vi "Swerve Drive.vi"(0 "X":dbl(slide) scale=-1.0..1.0, 1 "Rot. Point Y":dbl, 3 "Rot. Point X":dbl, 7 "Y":dbl(slide) scale=1.0..-1.0, 11 "Z":dbl(knob) scale=1.0..-1.0, 12 "Auto Controls":bool, 13 "Robot-Centric":bool) -> ()   [LabVIEW 2020]
uses:
  <vilib>/Rock Robotics/Network Tables/NT Write Boolean.vi
panel:
  in  "Robot Length":dbl=21.5
  in  "Robot Width":dbl=29.5
  # "SWERVE DRIVE\nVersion 3.1\n\nCory Lynch\nApple Pi Robotics\nTeam 2067"
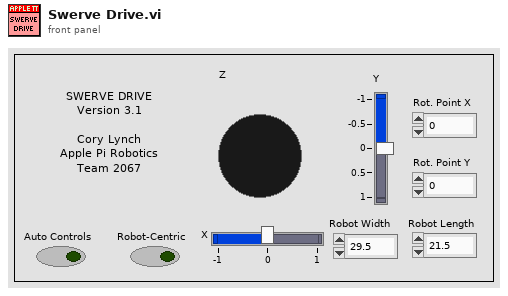
[diagram p1: front panel]
types:
  T1 = enum16{"Back Left", "Back Right", "Front Left", "Front Right"}
  T2 = cluster{"Yaw":dbl, "Roll":dbl, "Pitch":dbl, "Heading":dbl, "Fused Heading":dbl}
  T3 = typedef "WPI_MotorControlDeviceRef.ctl" = cluster{"DeviceStatus":errorcluster, "Type":T4, "PWM":cluster{"PWM Channel":T5, "DeadBand":T6}, "CAN":cluster{"Device Number":u8, "SetOutput VI Ref":variant, "GetOutput VI Ref":variant, "Enable VI Ref":variant, "Disable VI Ref":variant, "Data":variant}, "Invert":bool, "DIO PWM":cluster{"PWM \"Enable\" Channel":T5, "DIOChannel":T7, "PWM Rate":dbl}}
  T4 = typedef "WPI_MotorControlType.ctl" = enum16{"PWM", "CAN", "DIO PWM"}
  T5 = typedef "FPGA_DIOPWMChannel.ctl" = enum8{"PWM 0", "PWM 1", "PWM 2", "PWM 3", "PWM 4", "PWM 5", "PWM 6", "PWM 7", "PWM 8", "PWM 9", "PWM MXP 0", "PWM MXP 1", "PWM MXP 2", "PWM MXP 3", "PWM MXP 4", "PWM MXP 5", "PWM MXP 6", "PWM MXP 7", "PWM MXP 8", "PWM MXP 9", "Invalid"}
  T6 = typedef "WPI_PWMDeadband.ctl" = cluster{"Name":string, "maxPositivePwm":i32, "minPositivePwm":i32, "centerPwm":i32, "maxNegativePwm":i32, "minNegativePwm":i32, "angularRange":u16}
  T7 = typedef "FPGA_DIOChannel.ctl" = enum8{"DIO 0", "DIO 1", "DIO 2", "DIO 3", "DIO 4", "DIO 5", "DIO 6", "DIO 7", "DIO 8", "DIO 9", "DIO MXP 0", "DIO MXP 1", "DIO MXP 2", "DIO MXP 3", "DIO MXP 4", "DIO MXP 5", "DIO MXP 6", "DIO MXP 7", "DIO MXP 8", "DIO MXP 9", "DIO MXP 10", "DIO MXP 11", "DIO MXP 12", "DIO MXP 13", "DIO MXP 14", "DIO MXP 15", "SPI Port CS1", "SPI Port CS2", "SPI Port CS3", "SPI Port MISO", "SPI Port MOSI", "Invalid"}
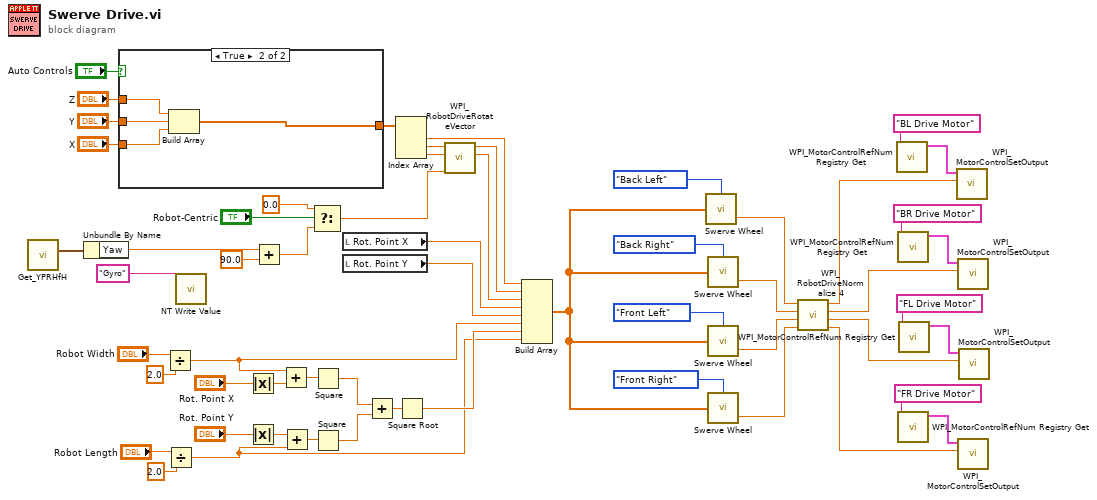
[diagram p0: block diagram]
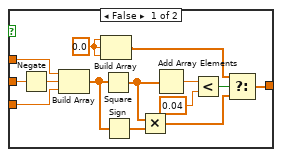
[diagram p2: hidden frame]
diagram:
  n1 = call <vilib>:"Get_YPRHfH.vi"() -> ("YRPHfH"=w6:T2)  [unwired: 11 in]
  n2 = Unbundle By Name(w6) -> ("Yaw"=w3:dbl)
  n3 = case shown="True" "Auto Controls" {
    tunnel: "Y" -> [w68 w74]
    tunnel: "X" -> [w62 w75]
    tunnel: "Z" -> [w58 w72]
    tunnel: [w59 w73] -> w14
    frame False {
      w66 = 0.0 ("element")
      n4 = Negate(x=w68) -> (-x=w61:dbl)
      n5 = Build Array(w58, w61, w62) -> (w65:dbl[])
      n6 = Build Array(w66, w66, w66) -> (w67:dbl[])
      n7 = Square(x=w65) -> (x^2=w63:dbl[])
      n8 = Sign(1:w65) -> (0:w64:dbl[])
      n9 = Multiply(x=w63, y=w64) -> (x*y=w60:dbl[])
      n10 = Add Array Elements(numeric array=w63) -> (sum=w71:dbl)
      n11 = Less?(x=w71, y=0.04 ("x")) -> (x < y?=w69:bool)
      n12 = Select(t=w67, s=w69, f=w60) -> (s? t:f=w59:dbl[])
    }
    frame True {
      n13 = Build Array(w72, w74, w75) -> (w73:dbl[])
    }
  }
  n14 = Divide(x="Robot Width", y=2.0) -> (x/y=w18:dbl)
  n15 = Divide(x="Robot Length", y=2.0) -> (x/y=w16:dbl)
  n16 = call-poly <vilib>:"NT Write Value.vi"("name"="Gyro" ("Name")) -> ()  [unwired: 10 in, 1 out]
  n17 = Absolute Value(x="Rot. Point X") -> (abs(x)=w36:dbl)
  n18 = Absolute Value(x="Rot. Point Y") -> (abs(x)=w34:dbl)
  n19 = Add(x=w3, y=90.0) -> (x+y=w2:dbl)
  n20 = Add(x=w18, y=w36) -> (x+y=w35:dbl)
  n21 = Add(x=w34, y=w16) -> (x+y=w33:dbl)
  n22 = Select(t=0.0, s="Robot-Centric", f=w2) -> (s? t:f=w10:dbl)
  n23 = Square(x=w35) -> (x^2=w31:dbl)
  n24 = Square(x=w33) -> (x^2=w32:dbl)
  n25 = local read "Rot. Point X"() -> (w20:dbl)
  n26 = local read "Rot. Point Y"() -> (w19:dbl)
  n27 = Add(x=w31, y=w32) -> (x+y=w30:dbl)
  n28 = Index Array(array=w14) -> (element #1=w9:dbl, element #2=w15:dbl, element #3=w23:dbl)  [unwired: 3 in]
  n29 = Square Root(x=w30) -> (sqrt(x)=w17:dbl)
  n30 = call <vilib>:"WPI_RobotDriveRotateVector.vi"("Angle"=w10, "X"=w23, "Y"=w15) -> ("X'"=w12:dbl, "Y'"=w8:dbl)  [unwired: 7 out]
  n31 = Build Array(w9, w8, w12, w20, w19, w18, w17, w16) -> (w13:dbl[])
  n32 = call "Swerve Wheel.vi"("Wheel"=T1."Back Left", "Inputs"=w13) -> ("Speed"=w54:dbl)  [unwired: 3 in]
  n33 = call "Swerve Wheel.vi"("Wheel"=T1."Back Right", "Inputs"=w13) -> ("Speed"=w53:dbl)  [unwired: 3 in]
  n34 = call "Swerve Wheel.vi"("Wheel"=T1."Front Left", "Inputs"=w13) -> ("Speed"=w52:dbl)  [unwired: 3 in]
  n35 = call "Swerve Wheel.vi"("Wheel"=T1."Front Right", "Inputs"=w13) -> ("Speed"=w51:dbl)  [unwired: 3 in]
  n36 = call <vilib>:"WPI_RobotDriveNormalize 4.vi"("D"=w51, "C"=w52, "B"=w53, "A"=w54) -> ("D'"=w38:dbl, "C'"=w39:dbl, "B'"=w40:dbl, "A'"=w41:dbl)
  n37 = call <vilib>:"WPI_MotorControlRefNum Registry Get.vi"("refnum name"="BL Drive Motor") -> ("MotorControlDevRef"=w49:T3)  [unwired: 9 in, 1 out]
  n38 = call <vilib>:"WPI_MotorControlRefNum Registry Get.vi"("refnum name"="BR Drive Motor") -> ("MotorControlDevRef"=w46:T3)  [unwired: 9 in, 1 out]
  n39 = call <vilib>:"WPI_MotorControlRefNum Registry Get.vi"("refnum name"="FR Drive Motor") -> ("MotorControlDevRef"=w42:T3)  [unwired: 9 in, 1 out]
  n40 = call <vilib>:"WPI_MotorControlRefNum Registry Get.vi"("refnum name"="FL Drive Motor") -> ("MotorControlDevRef"=w45:T3)  [unwired: 9 in, 1 out]
  n41 = call <vilib>:"WPI_MotorControlSetOutput.vi"("Output"=w41, "MotorControlDevRef"=w49) -> ()  [unwired: 7 in, 3 out]
  n42 = call <vilib>:"WPI_MotorControlSetOutput.vi"("Output"=w40, "MotorControlDevRef"=w46) -> ()  [unwired: 7 in, 3 out]
  n43 = call <vilib>:"WPI_MotorControlSetOutput.vi"("Output"=w38, "MotorControlDevRef"=w42) -> ()  [unwired: 7 in, 3 out]
  n44 = call <vilib>:"WPI_MotorControlSetOutput.vi"("Output"=w39, "MotorControlDevRef"=w45) -> ()  [unwired: 7 in, 3 out]
